vi "静态字段(Read).vi"() -> ()   [LabVIEW 2013]
uses:
  Math.lvclass
panel:
  out "Rand":dbl
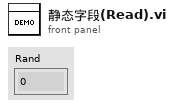
[diagram p1: front panel]
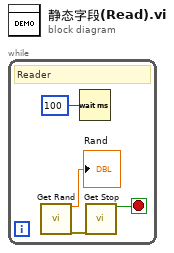
[diagram p0: block diagram]
diagram:
  n1 = while "While循环" {
    stop <- w2 stop-if-true
    # "Reader"
    n2 = call "Get Rand.vi"() -> ("Rand"=→"Rand":dbl, "error out"=w3:errorcluster)  [unwired: 18 in]
    n3 = Wait (ms)(milliseconds to wait=u32 100 ("等待时间（毫秒）")) -> ()  [unwired: 1 out]
    n4 = call "Get Stop.vi"("error in (no error)"=w3) -> ("Stop"=w2:bool)  [unwired: 17 in, 1 out]
  }
